vi "hotLotMSSQL.vi"() -> ()   [LabVIEW 2012]
uses:
  <vilib>/Utility/NIReport.llb/NI_report.lvclass
  <vilib>/addons/database/Connection.llb/DB Tools Open Connec (Path).vi
  <vilib>/addons/database/Connection.llb/Conn Execute.vi
  <vilib>/addons/database/Recordset.llb/Rec Fetch Integer Data (R).vi
  <vilib>/addons/database/Recordset.llb/Rec Destroy - Connection.vi
  Global1.vi
  <vilib>/addons/database/NI_Database_API.lvlib
  <vilib>/Utility/NIReport.llb/Excel/NI_Excel.lvclass
panel:
  out "data":string
  out "String":string
  out "error out 4":errorcluster
  out "Array":string[][](array[string])
  out "error out 3":errorcluster
  out "error out 2":errorcluster
  in  "Cluster":T1
  out "error out":errorcluster
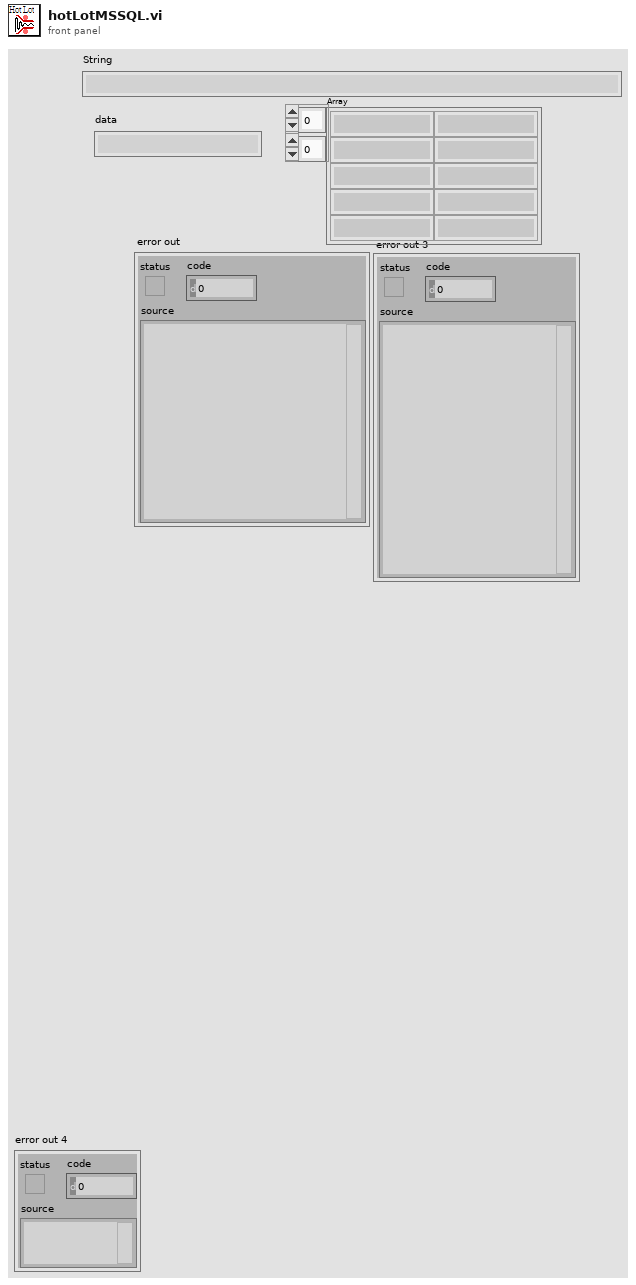
[diagram p1: front panel]
types:
  T1 = cluster{"type":string, "desc":string, "customer":string, "order":string, "cust_lot":string, "rc_no":string, "purpose":string, "device":string, "package":string, "qty":dbl, "step":string, "Due_date":string}
  T2 = enum16{"Standard Report", "HTML", "Word", "Excel"}
  T3 = typedef "NI_Database_API.lvlib/Conn ObjectReference.ctl" = refnum<k1>
  T4 = typedef "NI_Database_API.lvlib/Rec ObjectReference.ctl" = refnum<k1>
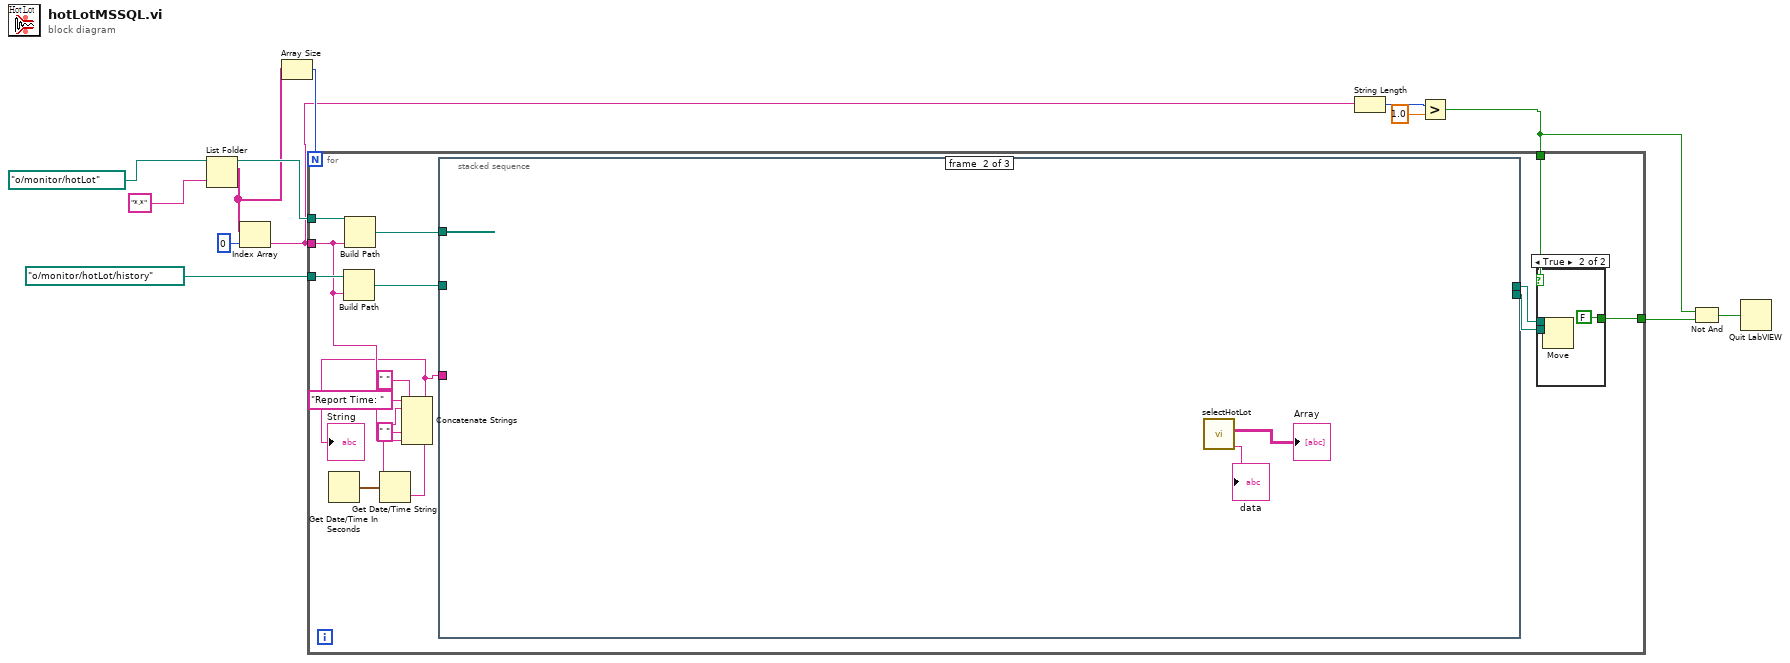
[diagram p0: block diagram]
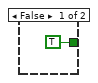
[diagram p2: hidden frame]
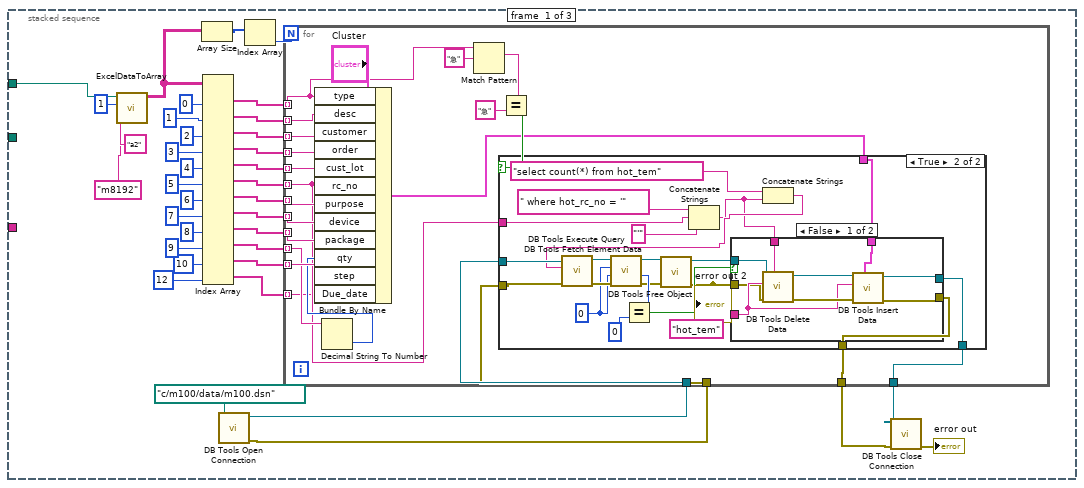
[diagram p3: hidden frame]
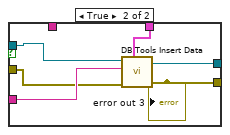
[diagram p5: hidden frame]
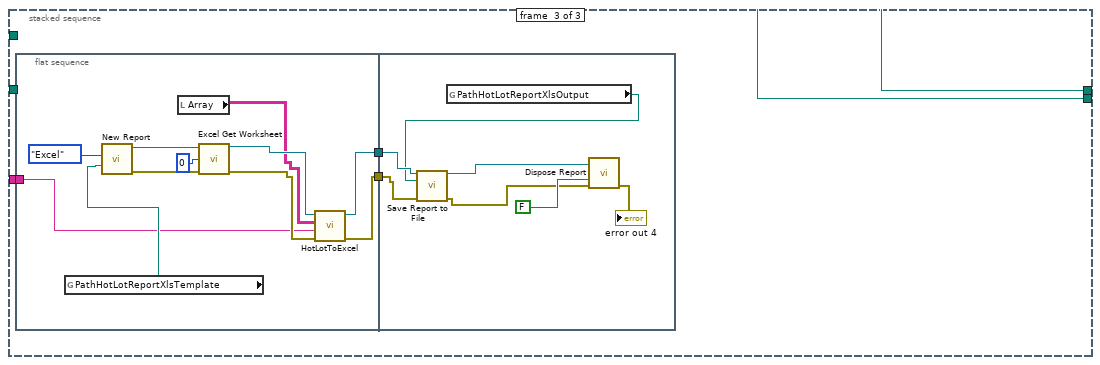
[diagram p6: hidden frame]
diagram:
  n1 = List Folder(path=path "o:/monitor/hotLot", pattern="*.*") -> (path out=w10:path, filenames=w9:string[])  [unwired: 2 in, 2 out]
  n2 = Index Array(array=w9, index=0) -> (element=w6:string)
  n3 = Array Size(array=w9) -> (size(s)=w12:i32)
  n4 = String Length(string=w6) -> (length=w4:i32)
  n5 = Greater?(x=w4, y=1.0) -> (0:w3:bool)
  n6 = for {
    N: w12 -> [_]
    tunnel: w6 -> [w16]
    tunnel: w10 -> [w29]
    tunnel: path "o:/monitor/hotLot/history" ("base path") -> [w27]
    tunnel: w3 -> [w23]
    tunnel: [w14] -> w2
    n7 = Get Date/Time In Seconds() -> (seconds since 1Jan1904=w22:timestamp)
    n8 = Build Path(base path=w27, name or relative path=w16) -> (appended path=w26:path)
    n9 = Build Path(base path=w29, name or relative path=w16) -> (appended path=w28:path)
    n10 = Get Date/Time String(seconds (now)=w22) -> (date string=w20:string, time string=w18:string)  [unwired: 2 in]
    n11 = Concatenate Strings("Report Time: " ("string"), w20, " " ("string"), w18, " " ("string"), w16) -> (w15:string)
    "String" <- w15
    n12 = stacked-sequence {
      tunnel: w28 -> [w36 _ w139]
      tunnel: w26 -> [_ _ w138]
      tunnel: [_ _ w139] -> w25
      tunnel: [_ _ w138] -> w24
      tunnel: w15 -> [_ _ w137]
      frame #0 {
        n13 = call "ExcelDataToArray.vi"("end cell"="m8192", "start cell"="a2", "sheet#"=1, "path"=w36) -> ("data"=w62:string[][])  [unwired: 6 in, 1 out]
        n14 = Array Size(array=w62) -> (size(s)=w66:i32[])
        n15 = Index Array(array=w62, index (col) #1=0 ("disabled index (col)"), index (col) #2=1 ("index (col)"), index (col) #3=2 ("index (col)"), index (col) #4=3 ("index (col)"), index (col) #5=4 ("index (col)"), index (col) #6=5 ("index (col)"), index (col) #7=6 ("index (col)"), index (col) #8=7 ("index (col)"), index (col) #9=8 ("index (col)"), index (col) #10=9 ("index (col)"), index (col) #11=10 ("index (col)"), index (col) #12=12 ("index (col)")) -> (element #1=w51:string[], element #2=w50:string[], element #3=w49:string[], element #4=w48:string[], element #5=w47:string[], element #6=w46:string[], element #7=w45:string[], element #8=w44:string[], element #9=w43:string[], element #10=w42:string[], element #11=w41:string[], element #12=w34:string[])  [unwired: 12 in]
        n16 = call-poly <vilib>:"DB Tools Open Connection.vi"("connection information"=path "c:/m100/data/m100.dsn") -> ("error out"=w39:errorcluster, "connection reference"=w40:T3)  [unwired: 7 in]
        n17 = Index Array(array=w66) -> (element=w65:i32)  [unwired: 1 in]
        n18 = for {
          N: w65 -> [_]
          tunnel: w51 -> [w73] mode=indexing
          tunnel: w50 -> [w91] mode=indexing
          tunnel: w49 -> [w90] mode=indexing
          tunnel: w48 -> [w89] mode=indexing
          tunnel: w47 -> [w88] mode=indexing
          tunnel: w46 -> [w77] mode=indexing
          tunnel: w45 -> [w84] mode=indexing
          tunnel: w44 -> [w85] mode=indexing
          tunnel: w43 -> [w86] mode=indexing
          tunnel: w42 -> [w79] mode=indexing
          tunnel: w41 -> [w87] mode=indexing
          tunnel: w40 -> [w81]
          tunnel: w39 -> [w80]
          tunnel: [w75] -> w38
          tunnel: [w76] -> w37
          tunnel: w34 -> [w74] mode=indexing
          n19 = Decimal String To Number(string=w79) -> (number=w78:i32)  [unwired: 2 in, 1 out]
          n20 = Bundle By Name(cluster="Cluster", "type"=w73, "desc"=w91, "customer"=w90, "order"=w89, "cust_lot"=w88, "rc_no"=w77, "purpose"=w84, "device"=w85, "package"=w86, "qty"=w78, "step"=w87, "Due_date"=w74) -> (w82:T1)
          n21 = Match Pattern(string=w73, regular expression="急") -> (match substring=w71:string)  [unwired: 1 in, 3 out]
          n22 = Equal?(x=w71, y="急") -> (x = y?=w83:bool)
          n23 = case shown="True" w83 {
            tunnel: w82 -> [_ w117]
            tunnel: w81 -> [w94 w116]
            tunnel: w80 -> [w95 w112]
            tunnel: w77 -> [_ w114]
            tunnel: [w95 w102] -> w76
            tunnel: [w94 w101] -> w75
            frame False {
            }
            frame True {
              w96 = 0
              n24 = Concatenate Strings(" where hot_rc_no = '" ("string"), w114, "'" ("string")) -> (w103:string)
              n25 = Concatenate Strings("select count(*) from hot_tem" ("string"), w103) -> (w104:string)
              n26 = call-poly <vilib>:"DB Tools Execute Query.vi"("error in (no error)"=w112, "SQL query"=w104, "connection reference"=w116) -> ("error out"=w111:errorcluster, "recordset reference"=w110:T4)  [unwired: 5 in]
              n27 = call-poly <vilib>:"DB Tools Fetch Element Data.vi"("error in (no error)"=w111, "type"=w96, "column index"=w96, "recordset reference"=w110) -> ("error out"=w100:errorcluster, "data"=w109:i32, "recordset reference out"=w99:T4)  [unwired: 3 in]
              n28 = Equal?(x=w109, y=0) -> (x = y?=w107:bool)
              n29 = call-poly <vilib>:"DB Tools Free Object.vi"("error in (no error)"=w100, "recordset reference"=w99) -> ("error out"=w97:errorcluster, "connection reference"=w98:T3)  [unwired: 8 in]
              "error out 2" <- w97
              n30 = case shown="False" w107 {
                tunnel: w117 -> [w122 w132]
                tunnel: [w121 w131] -> w101
                tunnel: [w120 w130] -> w102
                tunnel: "hot_tem" ("table") -> [w123 w129]
                tunnel: w103 -> [w126 _]
                tunnel: w98 -> [w119 w128]
                tunnel: w97 -> [w118 w127]
                frame False {
                  n31 = call <vilib>:"DB Tools Delete Data.vi"("condition"=w126, "error in (no error)"=w118, "table"=w123, "connection reference"=w119) -> ("error out"=w125:errorcluster, "connection reference out"=w124:T3)  [unwired: 6 in]
                  n32 = call <vilib>:"DB Tools Insert Data.vi"("data"=w122, "error in (no error)"=w125, "table"=w123, "connection reference"=w124) -> ("error out"=w120:errorcluster, "connection reference out"=w121:T3)  [unwired: 6 in]
                }
                frame True {
                  n33 = call <vilib>:"DB Tools Insert Data.vi"("data"=w132, "error in (no error)"=w127, "table"=w129, "connection reference"=w128) -> ("error out"=w130:errorcluster, "connection reference out"=w131:T3)  [unwired: 6 in]
                  "error out 3" <- w130
                }
              }
            }
          }
        }
        n34 = call <vilib>:"DB Tools Close Connection.vi"("error in (no error)"=w37, "connection reference"=w38) -> ("error out"=→"error out":errorcluster)  [unwired: 5 in]
      }
      frame #1 {
        n35 = call "selectHotLot.vi"() -> ("data"=→"data":string, "Array"=→"Array":string[][])  [unwired: 10 in]
      }
      frame #2 {
        n36 = flat-sequence {
          tunnel: w137 -> [w140]
          tunnel: [w143] -> w136
          tunnel: [w142] -> w135
          tunnel: w136 -> [w153]
          tunnel: w135 -> [w152]
          frame #0 {
            n37 = global read "Global1.vi" "PathHotLotReportXlsTemplate"() -> (w146:path)
            n38 = call <vilib>:"New Report.vi"("report type"=T2."Excel" ("Report Type"), "template (empty)"=w146) -> ("report out"=w149:refnum<class "NI_report.lvclass">, "error out"=w148:errorcluster)  [unwired: 12 in]
            n39 = local read "Array"() -> (w141:string[][])
            n40 = call <vilib>:"Excel Get Worksheet.vi"("report in"=w149, "worksheet index (0)"=0, "error in (no error)"=w148) -> ("report out"=w145:refnum<class "NI_report.lvclass">, "error out"=w144:errorcluster)  [unwired: 11 in]
            n41 = call "HotLotToExcel.vi"("error in (no error)"=w144, "Header"=w140, "Input"=w141, "report in"=w145) -> ("error out"=w142:errorcluster, "report out"=w143:refnum<class "NI_report.lvclass">)  [unwired: 6 in]
          }
          frame #1 {
            n42 = global read "Global1.vi" "PathHotLotReportXlsOutput"() -> (w151:path)
            n43 = call-dynamic "Save Report to File.vi"("report in"=w153, "report file path"=w151, "error in (no error)"=w152) -> ("report out"=w154:refnum<class "NI_report.lvclass">, "error out"=w155:errorcluster)  [unwired: 11 in]
            n44 = call-dynamic "Dispose Report.vi"("report in"=w154, "save changes? (F)"=FALSE, "error in (no error)"=w155) -> ("error out"=→"error out 4":errorcluster)  [unwired: 12 in]
          }
        }
      }
    }
    n45 = case shown="True" w23 {
      tunnel: w25 -> [_ w33]
      tunnel: w24 -> [_ w32]
      tunnel: [TRUE FALSE] -> w14
      frame False {
      }
      frame True {
        n46 = Move(source path=w33, 10:w32) -> ()  [unwired: 3 in, 3 out]
      }
    }
  }
  n47 = Not And(1:w2, 2:w3) -> (0:w1:bool)
  n48 = Quit LabVIEW(quit? (T)=w1) -> ()
